vi "Waiting for rising or falling edge of the signal START.vi"(8 "error in":errorcluster, 9 "Rising/Falling edge":bool, 10 "Variable name":string, 11 "UTP IO Session in":T1) -> (0 "error out":errorcluster, 3 "UTP IO Session out":T1)   [LabVIEW 2023, in "Actuators.lvlib"]
doc: "True for the Rising Edge\nFalse for the Falling Edge"
uses:
  Actuators.lvlib
  <vilib>/Noffz/UTP IO/UTP IO Library/Typedefs/Session Handle.ctl
  <vilib>/Noffz/UTP IO/UTP IO Library/UTP IO Pool Session.lvclass
  <vilib>/Noffz/UTP IO/UTP IO Library/methods/poly/plc/Read PLC Variable (Boolean).vi
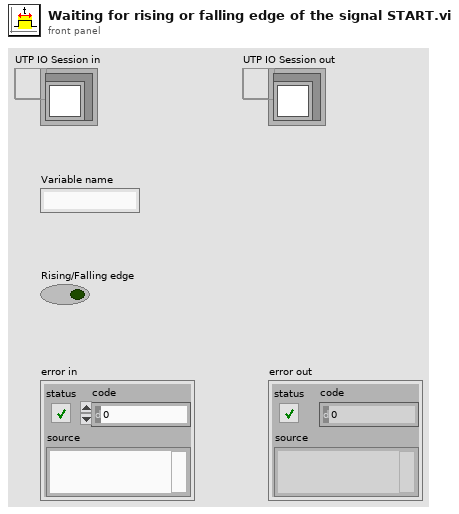
[diagram p1: front panel]
types:
  T1 = typedef "UTP IO Library.lvlib/UTP IO Pool Session.lvclass/Session Handle.ctl" = refnum<data-value>
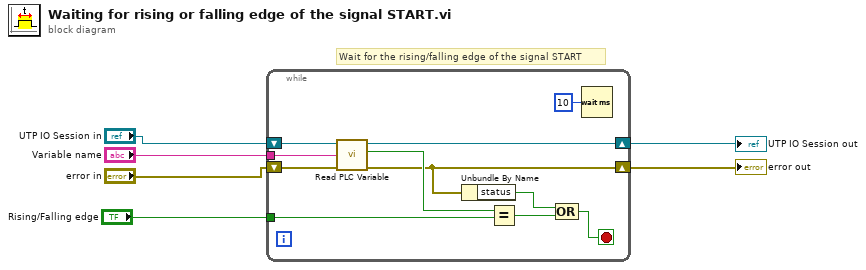
[diagram p0: block diagram]
diagram:
  # "Wait for the rising/falling edge of the signal START"
  n1 = while {
    tunnel: "Variable name" -> [w13]
    tunnel: "Rising/Falling edge" -> [w12]
    shift-right: [w15] -> w1
    shift-left: "UTP IO Session in" -> [w17]
    shift-right: [w11] -> w4
    shift-left: "error in" -> [w16]
    stop <- w9 stop-if-true
    n2 = call-poly <vilib>:"Read PLC Variable.vi"("error in (no error)"=w16, "variable name"=w13, "UTP IO Session in"=w17) -> ("error out"=w11:errorcluster, "value"=w14:bool, "UTP IO Session out"=w15:T1)  [unwired: 6 in]
    n3 = Unbundle By Name(w11) -> ("status"=w8:bool)
    n4 = Equal?(x=w14, y=w12) -> (x = y?=w7:bool)
    n5 = Compound Arithmetic op=OR(w8, w7) -> (w9:bool)
    n6 = Wait (ms)(milliseconds to wait=u32 10) -> ()  [unwired: 1 out]
  }
  "UTP IO Session out" <- w1
  "error out" <- w4
